vi "Write to Hardware.vi"(7 "Valid Triggers":bool, 8 "error in (no error)":errorcluster, 9 "Trigger Values":dbl[](array[numeric]), 10 "Values in":dbl[](array[numeric]), 11 "Tx Acyclic Execution Unit in":refnum<class "Tx Acyclic Labels Execution Unit.lvclass">) -> (0 "error out":errorcluster, 1 "Trigger Values out":dbl[](array[numeric]), 2 "Values out":dbl[](array[numeric]), 3 "Tx Acyclic Execution Unit out":refnum<class "Tx Acyclic Labels Execution Unit.lvclass">)   [LabVIEW 2020, in "AIM ARINC 429 Engine.lvlib" / "Implementation.lvlib" / "Tx Acyclic Labels Execution Unit.lvclass"]
uses:
  Tx Acyclic Labels Execution Unit.lvclass
  Hardware API/AIM ARINC 429 Hardware API.lvlib
  Execution Unit/Execution Unit.lvclass
  Custom Device/Custom Device.lvlib
  C:/Users/nitest/Desktop/Git 2020/niveristand-aim-arinc429-custom-device/Source/Custom Device Support/Engine/Implementation/Execution Unit/Execution Unit.lvclass
  C:/Users/nitest/Desktop/Git 2020/niveristand-aim-arinc429-custom-device/Source/Custom Device Support/Engine/Interfaces/Execution Unit/Execution Unit.lvclass
  C:/Users/nitest/Desktop/Git 2020/niveristand-aim-arinc429-custom-device/Source/Custom Device Support/Engine/Implementation/Tx Acyclic Labels Execution Unit/Tx Acyclic Labels Execution Unit.lvclass
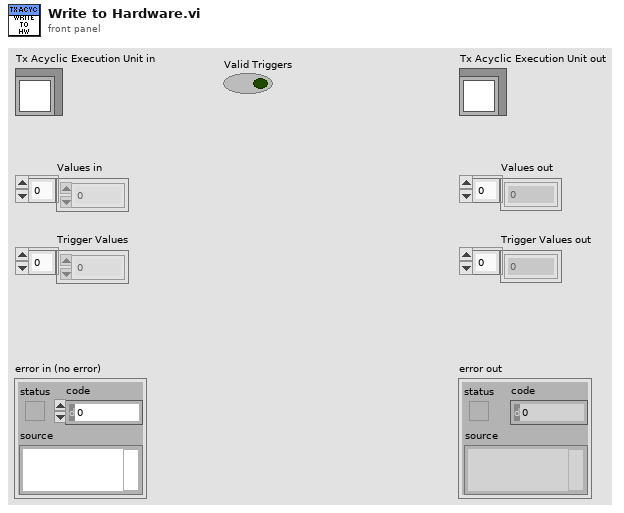
[diagram p1: front panel]
types:
  T1 = typedef "RT Hardware Channel Settings.ctl" = cluster{"channel #":u16, "channel handle":u64, "labels settings for RT":T2[], "speed":T10}
  T2 = typedef "RT Label Settings.ctl" = cluster{"Name":string, "xmlName":string, "label":T3, "transfer period":u32, "SDI_Enabled":bool, "SDI":u8, "parameter driver data":T4, "transfer type":T8, "has timestamp?":bool, "Label Disable/Trigger Channel Reference":T7, "Message Handle":u64, "Initialized?":bool, "Word Initial Raw Value":u32, "Label Timestamp Channel Data Reference":T9, "disabled":bool, "modified":bool}
  T3 = typedef "Label.ctl" = u8
  T4 = typedef "RT Parameters.ctl" = cluster{"parameter definitions":T5[], "Tx parameter refs":T7[]}
  T5 = typedef "Parameter Definition.ctl" = cluster{"start index":i32, "size":i32, "encoding":T6, "signed":bool, "scale multiplier":dbl, "scale offset":dbl, "default value":dbl}
  T6 = typedef "Encoding and Decoding.lvlib/Encoding.ctl" = enum16{"BNR", "BCD", "Discrete"}
  T7 = typedef "Custom Device API.lvlib/Custom Device Item Ref.ctl" = u64
  T8 = typedef "Transfer Type.ctl" = enum16{"Scheduled", "Acyclic", "Block", "Strobe"}
  T9 = typedef "Custom Device API.lvlib/Data Reference.ctl" = i32
  T10 = typedef "Transfer Speed.ctl" = enum16{"LO (12.5 kb/s)", "HI (100 kb/s)"}
  T11 = typedef "AIM ARINC 429 Hardware API.lvlib/Data Word with Trigger.ctl" = cluster{"Trigger":bool, "Data Word":u32}
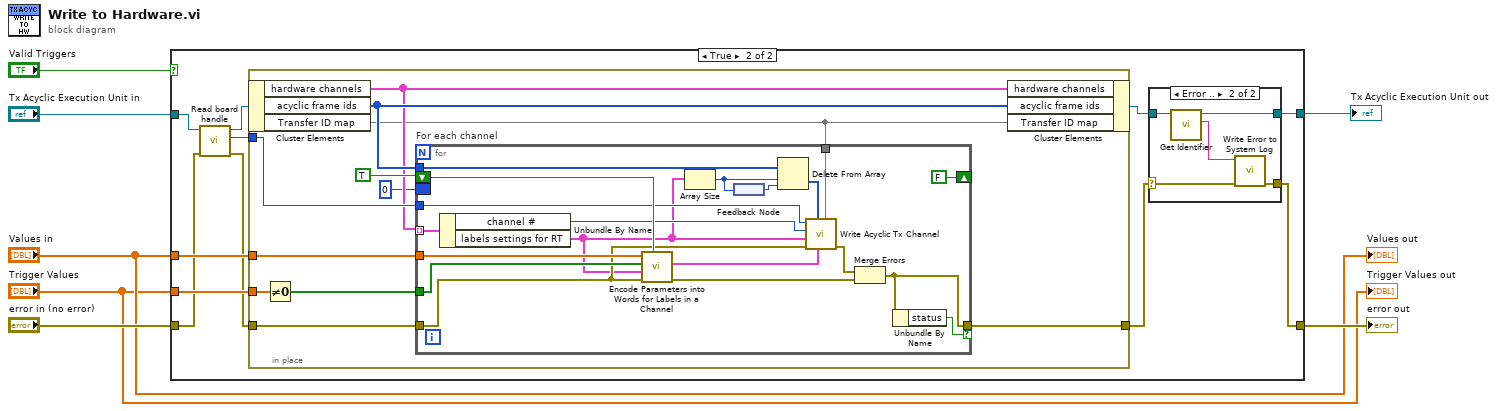
[diagram p0: block diagram]
diagram:
  n1 = case shown="True" "Valid Triggers" {
    tunnel: "Tx Acyclic Execution Unit in" -> [w9 w18]
    tunnel: [w9 w12] -> w5
    tunnel: "error in (no error)" -> [w8 w16]
    tunnel: [w8 w10] -> w3
    tunnel: "Values in" -> [_ w20]
    tunnel: "Trigger Values" -> [_ w19]
    frame False {
      # "if triggers are not valid, skip acyclic writes"
    }
    frame True {
      n2 = call "Read board handle.vi"("error in (no error)"=w16, "Execution Unit in"=w18) -> ("error out"=w15:errorcluster, "board handle"=w14:u8, "Execution Unit out"=w17:refnum<class "Tx Acyclic Labels Execution Unit.lvclass">)  [unwired: 7 in]
      n3 = in-place {
        in-place-border: w20 -> [w37]
        in-place-border: w19 -> [w38]
        in-place-border: w15 -> [w36]
        in-place-border: [w32] -> w11
        in-place-border: w14 -> [w33]
        n4 = in-place-cluster #1(w17) -> ("hardware channels"=w30:T1[], "acyclic frame ids"=w31:u32[], "Transfer ID map"=w28:map{u32, u32})
        n5 = Not Equal To 0?(x=w38) -> (x != 0?=w35:bool[])
        n6 = for "For each channel" {
          tunnel: w30 -> [w57] mode=indexing
          tunnel: w37 -> [w56]
          tunnel: w35 -> [w53]
          shift-right: [FALSE] -> _
          shift-left: TRUE -> [w54]
          tunnel: w33 -> [w50]
          border: 0 ("size(s)") -> [_]
          tunnel: w31 -> [w49]
          tunnel: w36 -> [w45]
          tunnel: [w42] -> w32 if=w41
          tunnel: w28 -> [w39]
          n7 = Unbundle By Name(w57) -> ("channel #"=w51:u16, "labels settings for RT"=w40:T2[])
          n8 = call "Encode Parameters into Words for Labels in a Channel.vi"("reset index"=w54, "error in (no error)"=w45, "labels settings for RT in"=w40, "Triggers in"=w53, "Parameter Values in"=w56) -> ("error out"=w43:errorcluster, "data with triggers out"=w52:T11[])  [unwired: 5 in]
          n9 = Array Size(array=w40) -> (size(s)=w46:i32)
          n10 = feedback-in #2(w46) -> ()
          n11 = feedback #2() -> (w47:i32)
          n12 = Delete From Array(array=w49, length=w46, index=w47) -> (deleted portion=w48:u32[])  [unwired: 1 out]
          n13 = call "Write Acyclic Tx Channel.vi"("Transfer ID map"=w39, "data with trigger in"=w52, "Acyclic Frame IDs in"=w48, "error in"=w45, "labels settings for RT"=w40, "channel number in"=w51, "board handle in"=w50) -> ("error out"=w44:errorcluster)  [unwired: 2 in, 2 out]
          n14 = Merge Errors(w44, w43) -> (w42:errorcluster)
          n15 = Unbundle By Name(w42) -> ("status"=w41:bool)
        }
        n16 = in-place-cluster #1("hardware channels"=w30, "acyclic frame ids"=w31, "Transfer ID map"=w28) -> (w13:refnum<class "Tx Acyclic Labels Execution Unit.lvclass">)
      }
      n17 = case shown="Error .." w11 {
        selector: w11 -> [w21 w24]
        tunnel: w13 -> [w22 w27]
        tunnel: [w22 w26] -> w12
        tunnel: [w21 w23] -> w10
        frame No Error {
        }
        frame Error {
          n18 = call-dynamic "Get Identifier.vi"("Execution Unit Implementation in"=w27) -> ("Identifier"=w25:string, "Execution Unit Implementation out"=w26:refnum<class "Tx Acyclic Labels Execution Unit.lvclass">)  [unwired: 8 in, 1 out]
          n19 = call "Write Error to System Log.vi"("error in"=w24, "identifier"=w25) -> ("error out"=w23:errorcluster)  [unwired: 9 in]
        }
      }
    }
  }
  "error out" <- w3
  "Tx Acyclic Execution Unit out" <- w5
  "Values out" <- "Values in"
  "Trigger Values out" <- "Trigger Values"
